vi "Set Menu Item Short Cut.vi"(7 "item tag":string, 8 "error in (no error)":errorcluster, 10 "short cut":T1, 11 "Menu in":refnum<class "Menu.lvclass">) -> (0 "error out":errorcluster, 3 "Menu out":refnum<class "Menu.lvclass">)   [LabVIEW 2021, in "Menu.lvlib" / "Menu.lvclass"]
uses:
  Menu.lvclass
  Menu.lvclass/Menu.ctl
  <vilib>/Utility/miscctls.llb/LVMapReplaceAction.ctl
  MenuItems.ctl
  <vilib>/Utility/miscctls.llb/LVMenuShortCut.ctl
  Picture2D/src/Picture/Image.lvclass
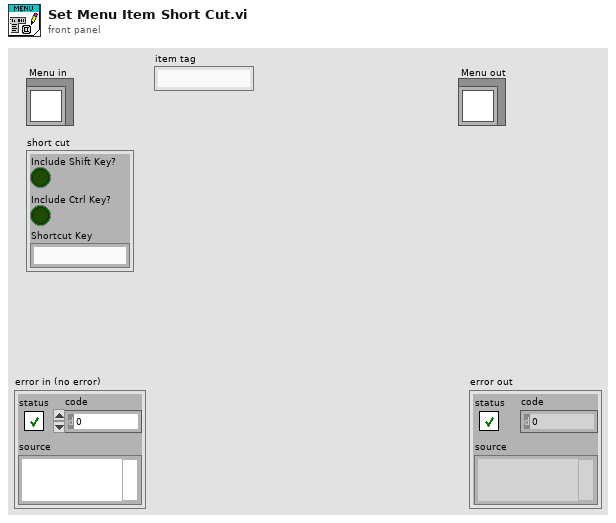
[diagram p1: front panel]
types:
  T1 = typedef "LVMenuShortCut.ctl" = cluster{"Include Shift Key?":bool, "Include Ctrl Key?":bool, "Shortcut Key":string}
  T2 = typedef "Menu.lvlib/Menu.lvclass/MenuItems.ctl" = cluster{"Item Name":string, "Short Cut":T1, "Checked":bool, "Enable":bool, "After item":string, "Item Tags":string[], "Item Names":string[], "Picture":refnum<class "Image.lvclass">, "Hilite Picture":refnum<class "Image.lvclass">, "Displayed":bool}
  T3 = typedef "LVMapReplaceAction.ctl" = enum32{"Modify Entry only if found", "Add or Modify Entry", "Delete Entry"}
  T4 = typedef "Menu.lvlib/Menu.lvclass/Data.ctl" = cluster{"MenuMap":map{string, T2}, "PictRef":refnum<vi>, "MenuSelectionEvent":refnum<user-event>, "TopMenuSpacing":i32, "MenuSpacing":i32, "CloseEvent":refnum<user-event>, "TR_ManageMenuRef":refnum<vi>, "MenuColors":T5, "RTMPath":path, "RTMVIReference":refnum<vi>, "RTMMenuReference":refnum<k9>, "CtlRef":refnum<vi>, "User-Specified Font":refnum<class "Font.lvclass">, "Desired Font":enum16{"User-specified Font", "Application Font", "System Font", "Dialog Font"}, "SubMenuIcon":T6, "SubMenuIconClosed":refnum<class "Picture2D.lvclass">, "SubMenuIconOpened":refnum<class "Picture2D.lvclass">}
  T5 = typedef "Menu.lvlib/Menu.lvclass/MenuColors.ctl" = cluster{"Text":refnum<class "Color.lvclass">, "HiliteText":refnum<class "Color.lvclass">, "Background":refnum<class "Color.lvclass">, "BorderColor":refnum<class "Color.lvclass">, "Hilite":refnum<class "Color.lvclass">}
  T6 = typedef "Menu.lvlib/Menu.lvclass/SubMenuIcon.ctl" = enum16{"LabVIEW", "Windows", "Custom"}
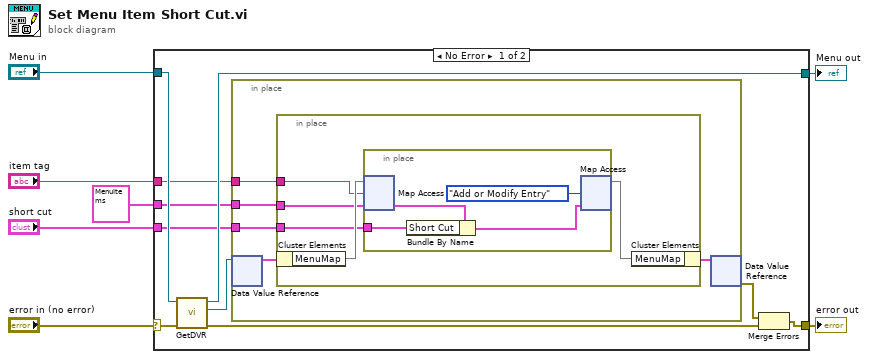
[diagram p0: block diagram]
diagram:
  n1 = case shown="No Error" "error in (no error)" {
    selector: "error in (no error)" -> [w17 w33]
    tunnel: [w10 w33] -> w6
    tunnel: [w15 w32] -> w4
    tunnel: "Menu in" -> [w14 w32]
    tunnel: "item tag" -> [w12 _]
    tunnel: "short cut" -> [w11 _]
    tunnel: T2 {"Item Name"="", "Short Cut"={"Include Shift Key?"=FALSE, "Include Ctrl Key?"=FALSE, "Shortcut Key"=""}, "Checked"=FALSE, "Enable"=TRUE, "After item"="", "Item Tags"=[], "Item Names"=[], "Picture"=refnum, "Hilite Picture"=refnum, "Displayed"=FALSE} ("Menu") -> [w8 _]
    frame No Error {
      n2 = call "GetDVR.vi"("error in (no error)"=w17, "Menu in"=w14) -> ("error out"=w16:errorcluster, "DVR"=w13:refnum<data-value>, "Menu out"=w15:refnum<class "Menu.lvclass">)  [unwired: 7 in]
      n3 = in-place {
        in-place-border: w12 -> [w21]
        in-place-border: w11 -> [w19]
        in-place-border: w8 -> [w18]
        n4 = in-place-dvr #1(w13) -> (w22:T4)  [unwired: 1 out]
        n5 = in-place {
          in-place-border: w21 -> [w26]
          in-place-border: w18 -> [w24]
          in-place-border: w19 -> [w23]
          n6 = in-place-cluster #2(w22) -> ("MenuMap"=w27:map{string, T2})
          n7 = in-place {
            in-place-border: w23 -> [w28]
            n8 = in-place-map #3(w27, w26, w24) -> (w30:T2)  [unwired: 1 out]
            n9 = Bundle By Name(cluster=w30, "Short Cut"=w28) -> (w29:T2)
            n10 = in-place-map #3(w29, LVMapReplaceAction."Add or Modify Entry" ("action")) -> (w25:map{string, T2})  [unwired: 2 out]
          }
          n11 = in-place-cluster #2("MenuMap"=w25) -> (w20:T4)
        }
        n12 = in-place-dvr #1(w20) -> (w9:errorcluster)  [unwired: 1 out]
      }
      n13 = Merge Errors(w9, w16) -> (w10:errorcluster)
    }
    frame Error {
    }
  }
  "error out" <- w6
  "Menu out" <- w4
